vi "GetType.vi"(8 "error in (no error)":errorcluster, 11 "Update_Moving Msg":refnum<class "Update_Moving Msg.lvclass">) -> (0 "error out":errorcluster, 2 "Data Sample":variant, 3 "Update_Moving Msg":refnum<class "Update_Moving Msg.lvclass">)   [LabVIEW 2015, in "CS++Motor.lvlib" / "Update_Moving Msg.lvclass"]
uses:
  Update_Moving Msg.lvclass
  Update_Moving Msg.lvclass/Update_Moving Msg.ctl
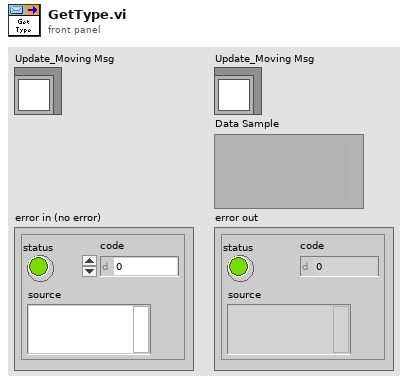
[diagram p1: front panel]
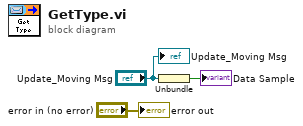
[diagram p0: block diagram]
diagram:
  n1 = Unbundle("Update_Moving Msg") -> (→"Data Sample":bool)
  "error out" <- "error in (no error)"
  "Update_Moving Msg" <- "Update_Moving Msg"
